vi "cRIO_Host_Cluster_Read_OldMethod_Benchmark.vi"() -> ()   [LabVIEW 2018]
uses:
  TypeDefs/Simple cluster.ctl
  <vilib>/addons/FPGA Advanced Session Resources/LVFPGA Adv Session Resources/OpenByNameSubVI.vi
  <vilib>/rvi/interface/common/dynamic/niFpgaEscapeDelimiterAndNull.vi
  <vilib>/Utility/error.llb/Error Cluster From Error Code.vi
  <vilib>/rvi/errors/niLvFpgaAdjustHostInterfaceError.vi
  <vilib>/FPGAPlugInAG/Dynamic/niLvFpga_Close_Dynamic.vi
  <vilib>/addons/FPGA Advanced Session Resources/LVFPGA Adv Session Resources/OpenByName.xnode
  <vilib>/rvi/interface/nirviReadWriteControl/nirviReadWriteControl.xnode
  <vilib>/rvi/interface/nirviCloseFPGA/nirviCloseFPGA.xnode
  <vilib>/addons/FPGA Advanced Session Resources/LVFPGA Adv Session Resources/LVFPGAAdvSessionResources.lvlib
  NiFpgaLv.dll
  <vilib>/rvi/interface/Simulation/niFpgaSimulationCallBeginRW.vi
panel:
  out "Array":T1(array[cluster])
  out "error out":errorcluster
  out "Execution time (s)":dbl
  # "Recorded time"
  # "3.37551E-5"
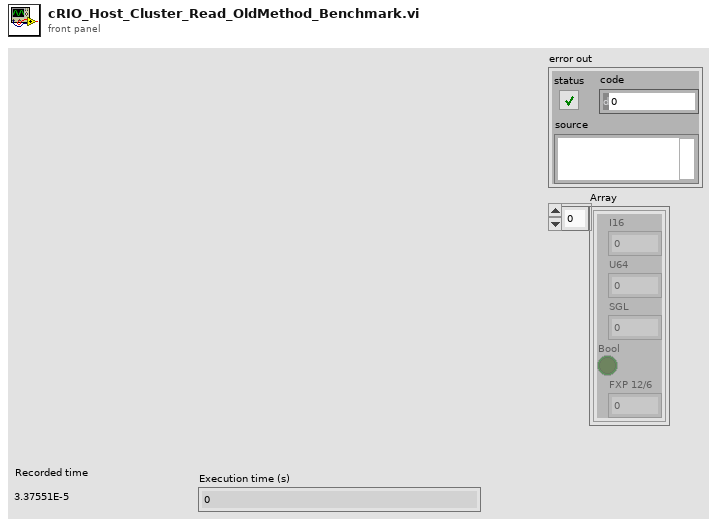
[diagram p1: front panel]
types:
  T1 = cluster{"I16":i16, "U64":u64, "SGL":sgl, "Bool":bool, "FXP 12/6":fxp<+/-,12,6>}[]
  T2 = typedef "Simple cluster.ctl" = cluster{"I16":i16, "U64":u64, "SGL":sgl, "Bool":bool, "FXP 12/6":fxp<+/-,12,6>}
  T3 = cluster{"I16":i16, "U64":u64, "SGL":sgl, "Bool":bool, "FXP 12/6":fxp<+/-,12,6>}
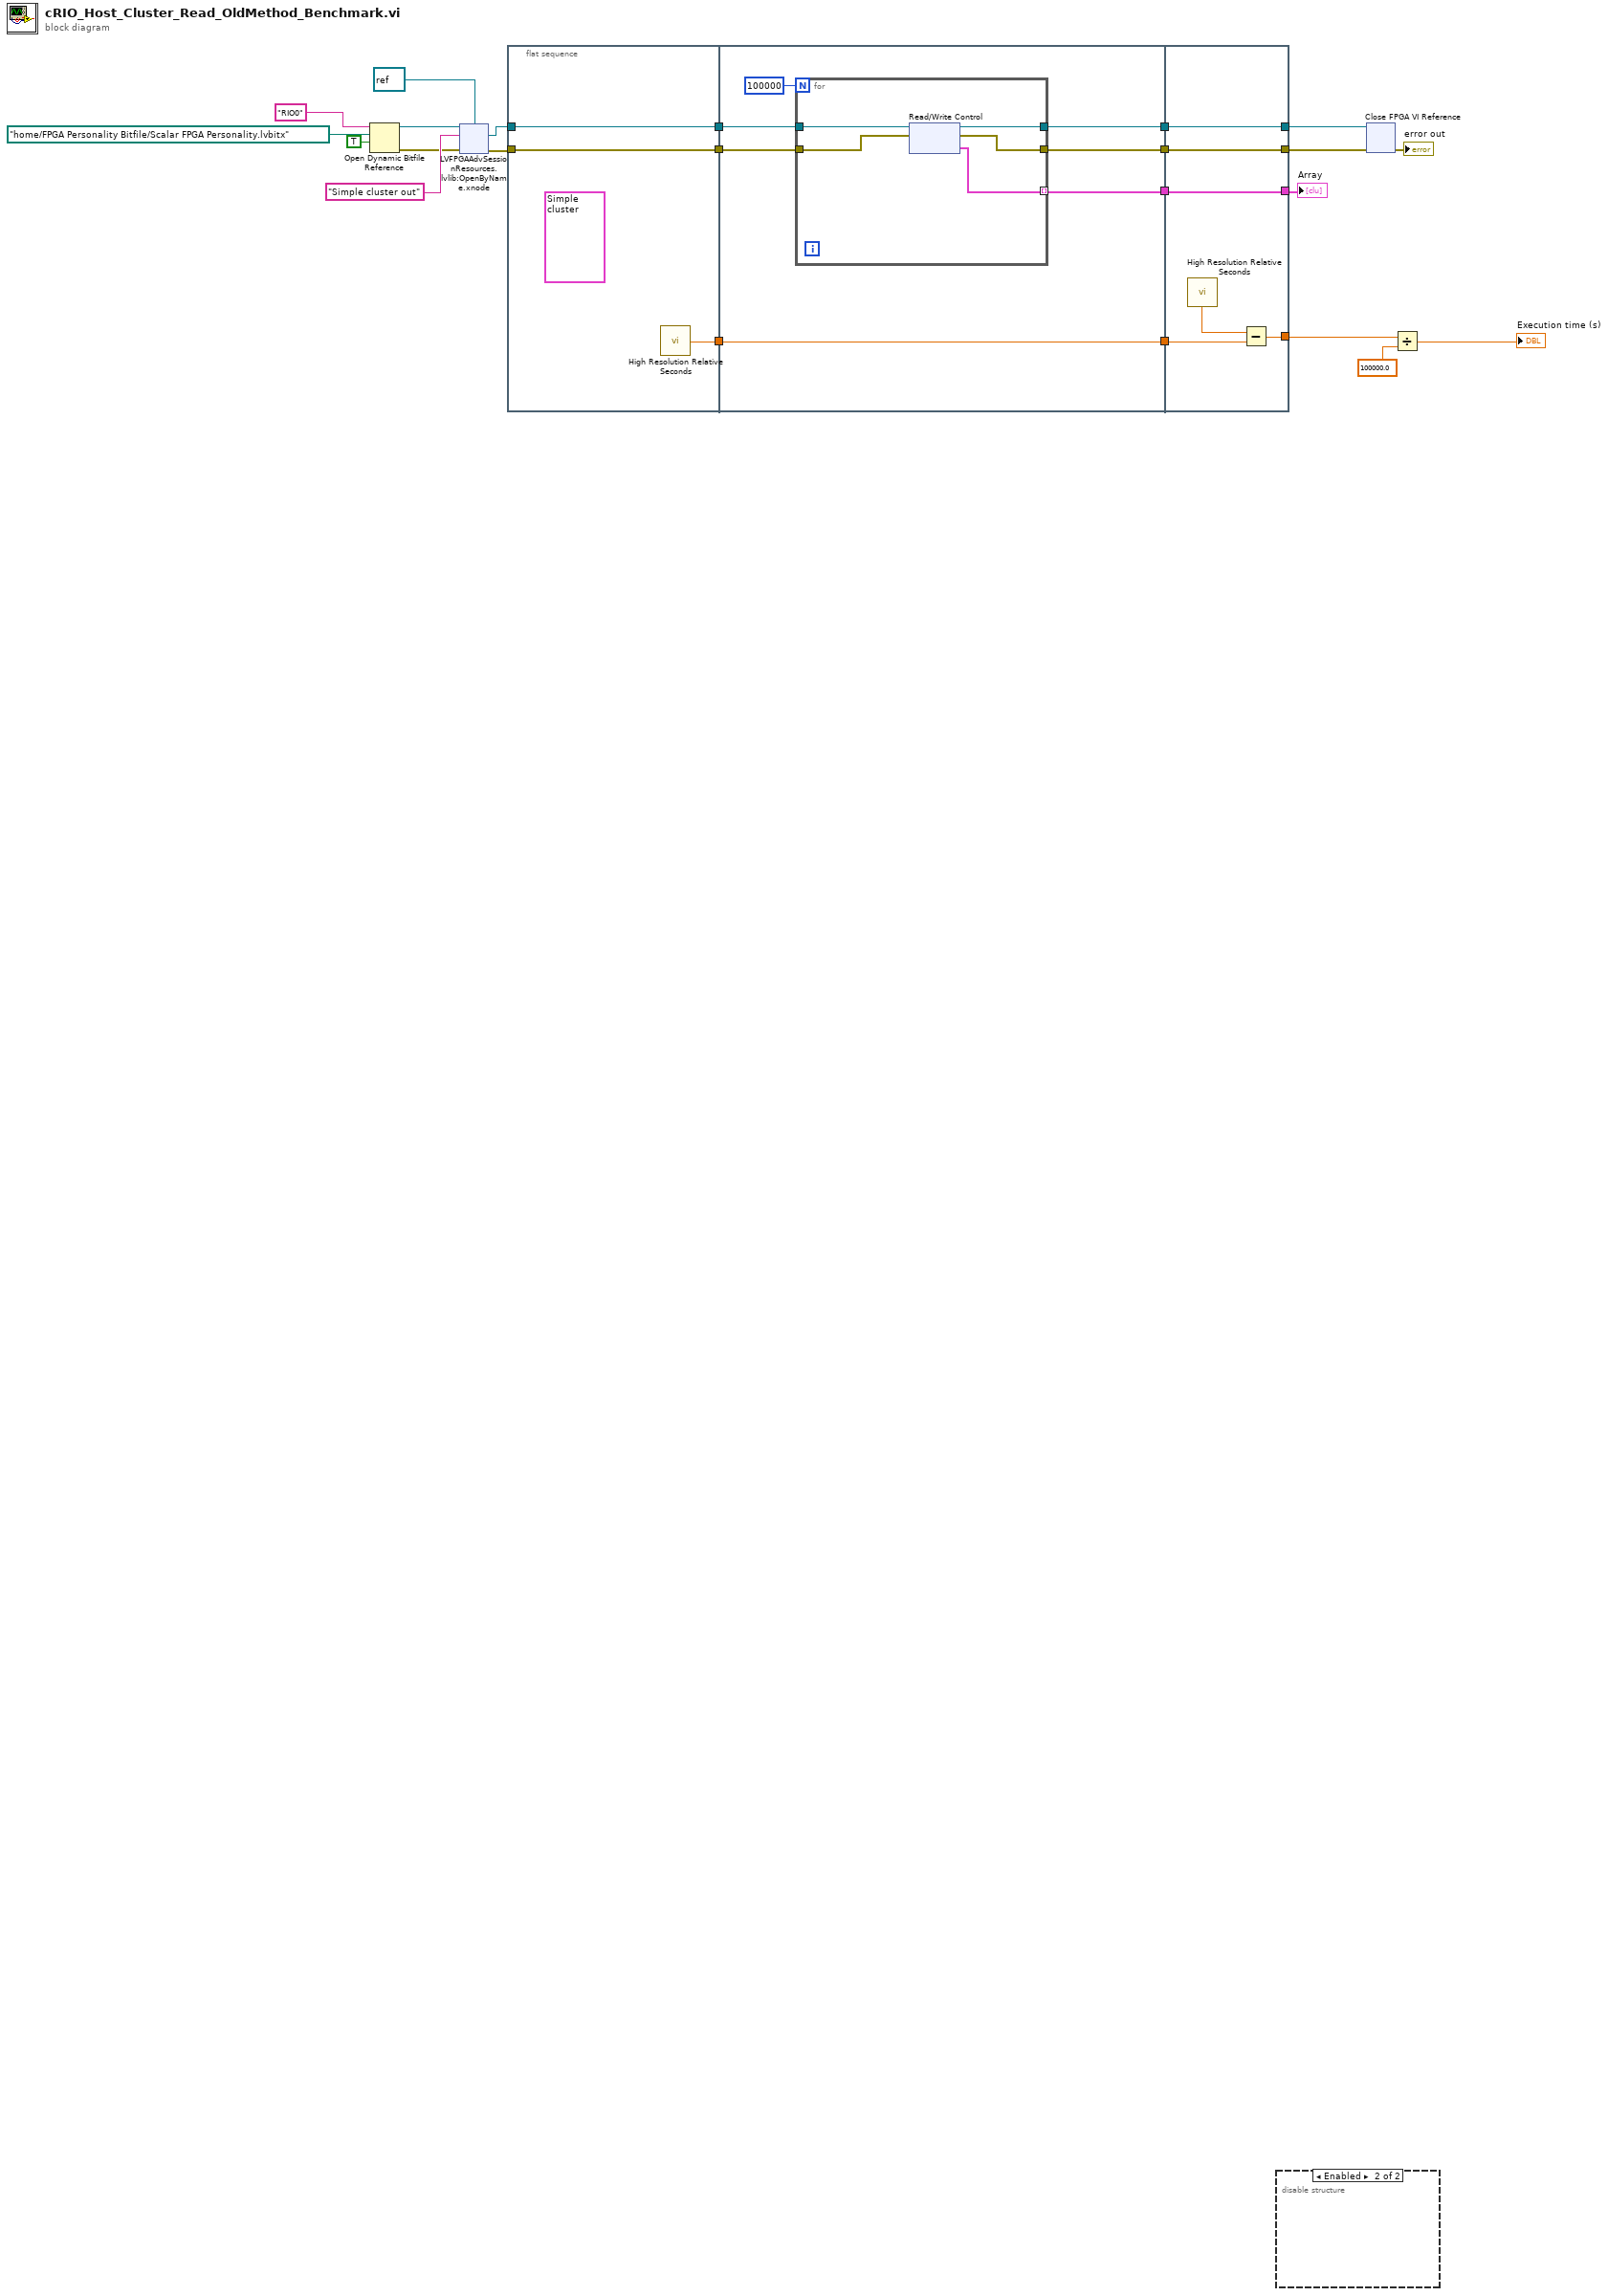
[diagram p0: block diagram]
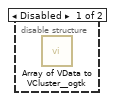
[diagram p2: hidden frame]
diagram:
  n1 = Open Dynamic Bitfile Reference(0:"RIO0" ("Device address"), 1:path "/home/FPGA Personality Bitfile/Scalar FPGA Personality.lvbitx" ("Bitfile path"), 2:TRUE ("Run When Loaded")) -> (5:w8:refnum<k20>, 8:w6:errorcluster)  [unwired: 2 in]
  n2 = xnode "LVFPGAAdvSessionResources.lvlib:OpenByName.xnode"("FPGA VI Reference in"=w8, "Resource name in"="Simple cluster out", "Single resource reference type in"=refnum<k20> refnum ("Type"), "Error in"=w6) -> ("Single resource reference out"=w4:refnum<k20>, "Error out"=w5:errorcluster)  [unwired: 1 out]
  n3 = flat-sequence {
    tunnel: [w26] -> w22
    tunnel: w4 -> [w25]
    tunnel: [w25] -> w15
    tunnel: [w24] -> w14
    tunnel: w5 -> [w24]
    tunnel: [w32] -> w23
    tunnel: w22 -> [w32]
    tunnel: w15 -> [w31]
    tunnel: w14 -> [w30]
    tunnel: [w29] -> w13
    tunnel: [w28] -> w12
    tunnel: [w27] -> w2
    tunnel: w23 -> [w43]
    tunnel: [w42] -> w21
    tunnel: w13 -> [w40]
    tunnel: w12 -> [w41]
    tunnel: [w41] -> w11
    tunnel: [w40] -> w10
    tunnel: [w39] -> w1
    tunnel: w2 -> [w39]
    frame #0 {
      (unwired) T2 {"I16"=1231, "U64"=213123, "SGL"=1.0, "Bool"=TRUE, "FXP 12/6"=31.984375} ("Simple Cluster")
      n4 = call <vilib>:"High Resolution Relative Seconds.vi"() -> ("relative seconds"=w26:dbl)
    }
    frame #1 {
      n5 = for {
        N: 100000 -> [_]
        tunnel: w31 -> [w38]
        tunnel: w30 -> [w37]
        tunnel: [w36] -> w29
        tunnel: [w35] -> w28
        tunnel: [w34] -> w27 mode=indexing
        n6 = xnode "Read/Write Control"("FPGA VI Reference In"=w38, "error in"=w37) -> ("FPGA VI Reference Out"=w35:refnum<k20>, "error out"=w36:errorcluster, "Value"=w34:T3)
      }
    }
    frame #2 {
      n7 = call <vilib>:"High Resolution Relative Seconds.vi"() -> ("relative seconds"=w44:dbl)
      n8 = Subtract(x=w44, y=w43) -> (x-y=w42:dbl)
    }
  }
  n9 = disable-structure shown="Enabled" {
    frame Disabled {
      n10 = call <userlib>:"Array of VData to VCluster__ogtk.vi"() -> ()  [unwired: 10 in, 2 out]
    }
    frame Enabled {
    }
  }
  n11 = xnode "Close FPGA VI Reference"("FPGA VI Reference In"=w11, "error in"=w10) -> ("error out"=→"error out":errorcluster)
  n12 = Divide(x=w21, y=100000.0) -> (x/y=→"Execution time (s)":dbl)
  "Array" <- w1
